vi "calcNewOutputs.vi"(8 "error in (no error)":errorcluster, 11 "Model in":refnum<class "Model.lvclass">) -> (0 "error out":errorcluster, 3 "Model out":refnum<class "Model.lvclass">)   [LabVIEW 2013, in "Model.lvclass"]
uses:
  Model.lvclass
  StreamingDataAlgorithms/StreamingDataAlgorithm/StreamingDataAlgorithm.lvclass
  <userlib>/Common/ILC/ILC/ILC.lvclass
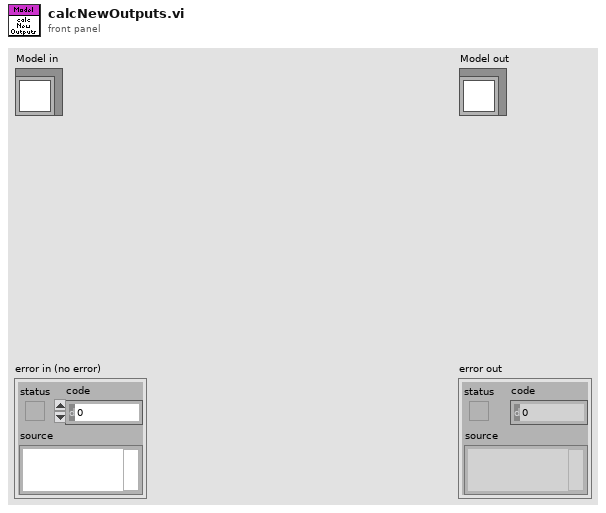
[diagram p1: front panel]
types:
  T1 = typedef "ILCCommon.lvlib/ILCTypedefs.lvlib/OutputData.ctl" = cluster{"Step & Direction":i16, "Blower RPM":u8, "PWM (SSR)":u8, "Ch1":u16, "Ch2":u16, "Ch3":u16, "Ch4":u16}
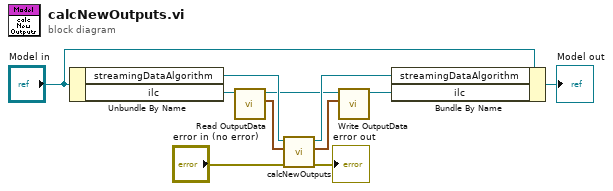
[diagram p0: block diagram]
diagram:
  n1 = Unbundle By Name("Model in") -> ("streamingDataAlgorithm"=w11:refnum<class "StreamingDataAlgorithm.lvclass">, "ilc"=w5:refnum<class "ILC.lvclass">)
  n2 = call <userlib>:"Read OutputData.vi"("ILC in"=w5) -> ("OutputData"=w4:T1, "ILC out"=w3:refnum<class "ILC.lvclass">)  [unwired: 9 in]
  n3 = call-dynamic "calcNewOutputs.vi"("error in (no error)"="error in (no error)", "outputData"=w4, "StreamingDataAlgorithm in"=w11) -> ("error out"=→"error out":errorcluster, "outputData 2"=w2:T1, "StreamingDataAlgorithm out"=w8:refnum<class "StreamingDataAlgorithm.lvclass">)  [unwired: 6 in]
  n4 = call <userlib>:"Write OutputData.vi"("OutputData"=w2, "ILC in"=w3) -> ("ILC out"=w1:refnum<class "ILC.lvclass">)  [unwired: 9 in]
  n5 = Bundle By Name(cluster="Model in", "streamingDataAlgorithm"=w8, "ilc"=w1) -> (→"Model out":refnum<class "Model.lvclass">)
